vi "MARS_SiPM_Data_Analysis.vi"() -> ()   [LabVIEW 2015]
uses:
  <vilib>/Utility/tdmsutil.llb/fileViewerConfigData.ctl
  Data_Analysis_subvis/ESA_Data_Analysis_Global_VIs.vi
  <vilib>/Analysis/NI_AALPro.lvlib
panel:
  in  "Add Chs":bool
  in  "Offset":dbl=-7.5e-05 step=1e-05 format="%#.3p"
  in  "Discr. Slope":dbl=3.07 min=0.0 step=0.1 format="%#.3p"
  out "Indicator":bool
  in  "Listbox":i32[](listbox) caption="File Name"
  in  "Contents sel":bool
  in  "Sim. Analysis":bool
  in  "Tab Sel 2":enum32{"Radio Selection 1", "Radio Selection 2"}(radio)
  in  "Analysis tab":enum32{"Analysis", "Spectrum"}(tab)
  out "Intensity Graph":u32[][](graph)
  out "Histogram":u32[](graph)
  in  "Graph sel":bool=TRUE
  out "Scatter Plot":cluster{"Array":dbl[], "Array":dbl[]}[](graph)
  in  "File Vs Discr":bool
  in  "PeakVs Integral":bool
  out "Spectrum":T1(graph)
  in  "# bins":i32=256
  in  "Max":dbl=0.2 format="%#.3p"
  in  "Min":dbl format="%#.3p"
  out "Nb of Neutron Counts":i32
  out "Nb of Gamma Counts":i32
  out "Total Counts":i32
  in  "Tab Sel":T2(radio)
  in  "Data tab":enum32{"Raw", "Filtered", "Properties"}(tab)
  out "Boolean 2":bool
  out "Boolean":bool
  in  "Nb of Samples as Offset":i32=50
  in  "Display sel":bool
  out "SiPM Waveform":waveform(dbl)[](graph)
  out "Total Int.":dbl caption="Total Integration Duration (s)" format="%#.3p"
  out "Tail Int.":dbl caption="Tail Integration Duration (s)" format="%#.3p"
  in  "Nb of Samples to Display":i32=50
  out "T3b (s)":dbl format="%#.3p"
  out "T2b (s)":dbl format="%#.3p"
  out "T1b (s)":dbl format="%#.3p"
  out "T3a (s)":dbl format="%#.3p"
  out "T2a (s)":dbl format="%#.3p"
  out "T1a (s)":dbl format="%#.3p"
  out "Table":string[][](table)
  in  "Std Dev 3":dbl=0.005 format="%0.2f"
  in  "Std Dev 2":dbl=0.04 format="%0.2f"
  in  "Graph resolution":dbl=5.0
  in  "Com. std dev":dbl=0.4 format="%0.2f"
  in  "Create Graph":bool
  in  "Nb of smpls":i32=10 min=0 max=50000
  in  "Stop Button":bool
  in  "Open Button":bool
  out "Spectrum Data":T3
  out "Integral Spectrum":dbl[][](array[numeric])
  out "Bins cluster":cluster{"Max":dbl, "Min":dbl, "# bins":i32}
  out "Discr. Slope":cluster{"Array":dbl[], "Array":dbl[]}
  out "Scatter Data":cluster{"Array":dbl[], "Array":dbl[]}
  out "Nb of Channels in Group":i32
  out "Array 2":dbl[](array[numeric])
  out "Array 1":dbl[](array[numeric])
  out "dt":dbl
  out "Total Integral":dbl[](array[numeric])
  out "Tail Integral":dbl[](array[numeric])
  out "group names":string[](array[string])
  out "tdms file out":refnum<k34>
  in  "File contents":string[](tree)
  # "MARS  SiPM Characterization"
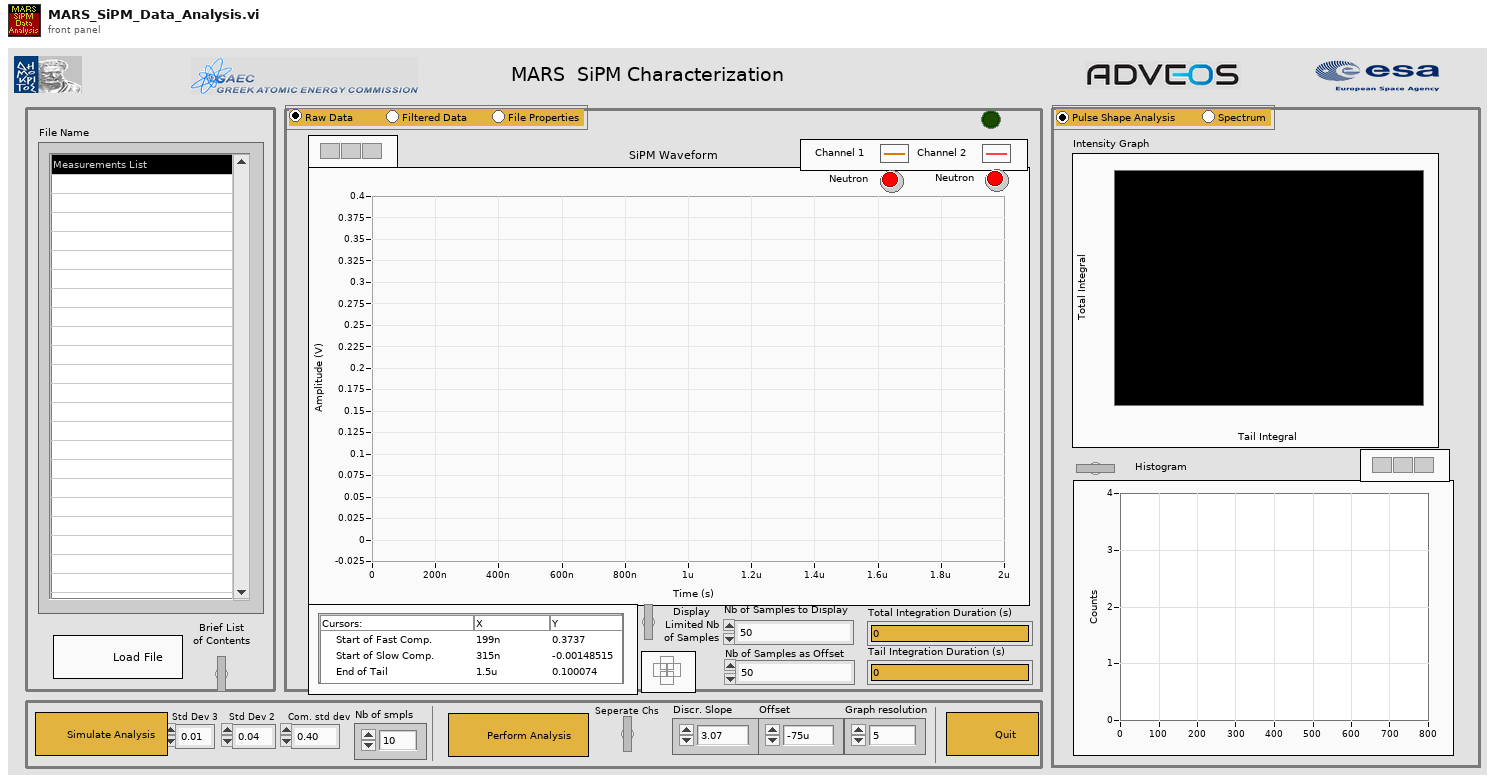
[diagram p1: front panel]
types:
  T1 = cluster{"X Values":dbl[], "Histogram: h(x)":i32[]}[]
  T2 = enum32{"Radio Selection 1", "Radio Selection 2", "Radio Selection 3"}
  T3 = cluster{"Gamma Spectrum":dbl[], "Gamma Integral":dbl[], "Neutron Spectrum":dbl[], "Neutron Integral":dbl[]}
  T4 = typedef "fileViewerConfigData.ctl" = cluster{"Show all (table)":bool, "Show all (graph)":bool, "limit (table)":u64, "limit (graph)":u64, "no show":bool, "start (table)":u64, "start (graph)":u64}
  T5 = enum16{"open", "open or create", "create or replace", "create", "open (read-only)"}
  T6 = cluster{"Cursor.Cursor X":dbl, "Cursor.Cursor Y":dbl, "Cursor.Cursor X":dbl, "Cursor.Cursor Y":dbl}
  T7 = cluster{"X Values":dbl[], "Histogram: h(x)":i32[]}
  T8 = cluster{"Numeric Control":i32, "Numeric Control":i32, "Numeric Control":i32}
  T9 = cluster{"Scatter Plot":cluster{"Array":dbl[], "Array":dbl[]}, "Intensity graph":u32[][], "Histogram":u32[]}
  T10 = cluster{"Tail Integral":dbl[], "Total Integral":dbl[]}
  T11 = cluster{"Tail Integral":dbl[], "Total Integral":dbl[]}[]
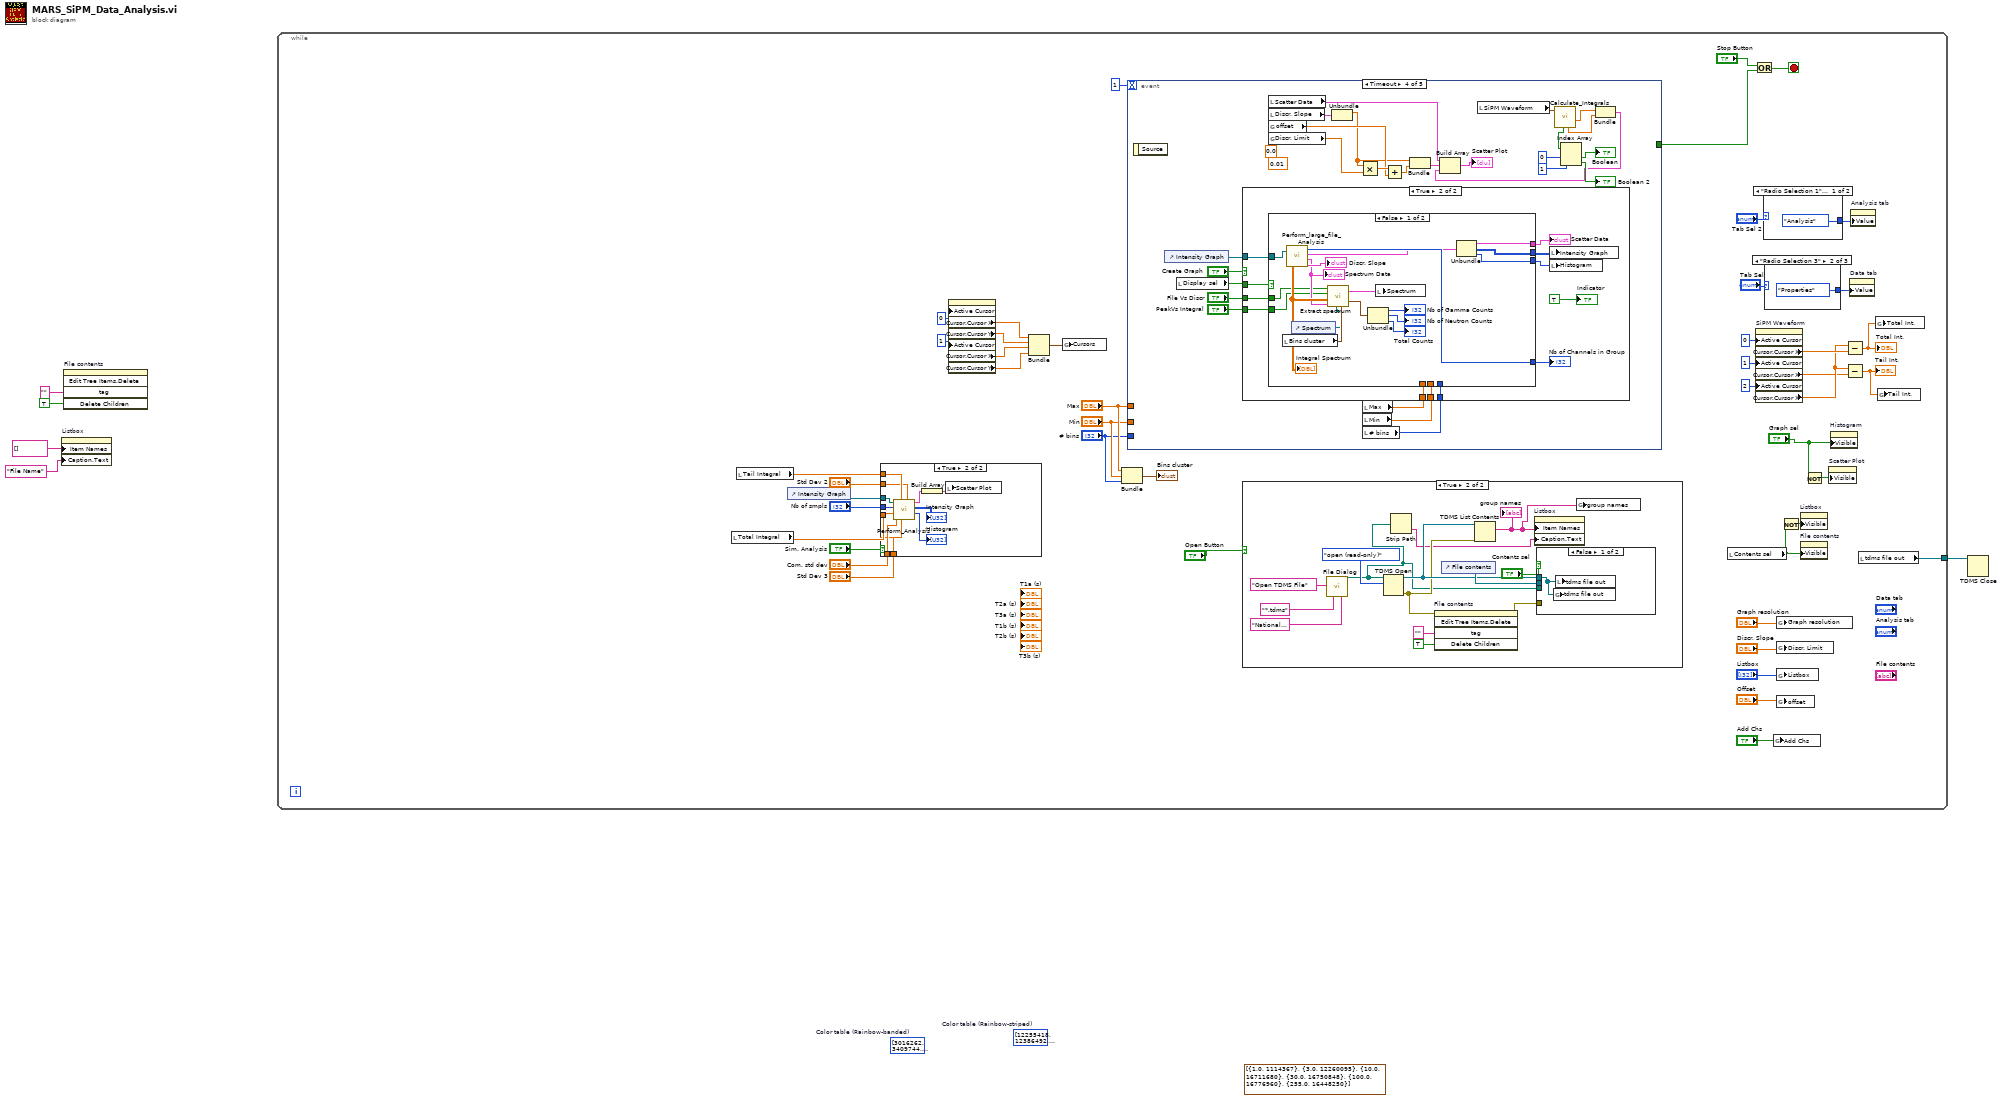
[diagram p0: block diagram]
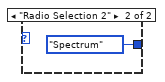
[diagram p2: hidden frame]
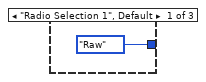
[diagram p3: hidden frame]
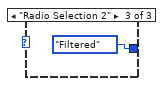
[diagram p4: hidden frame]
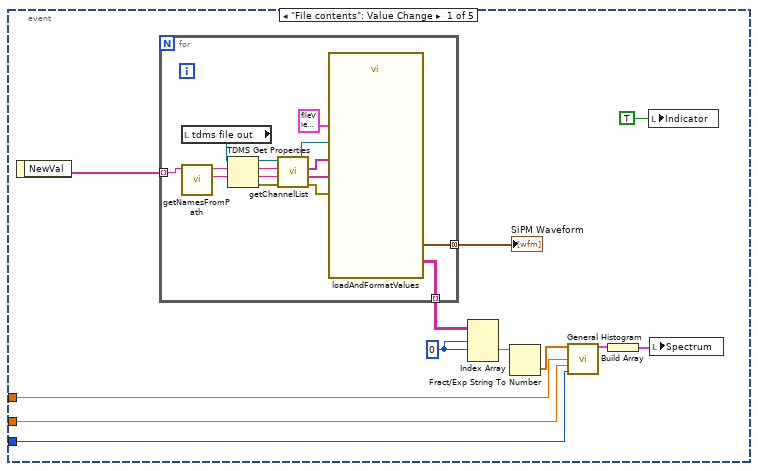
[diagram p6: hidden frame]
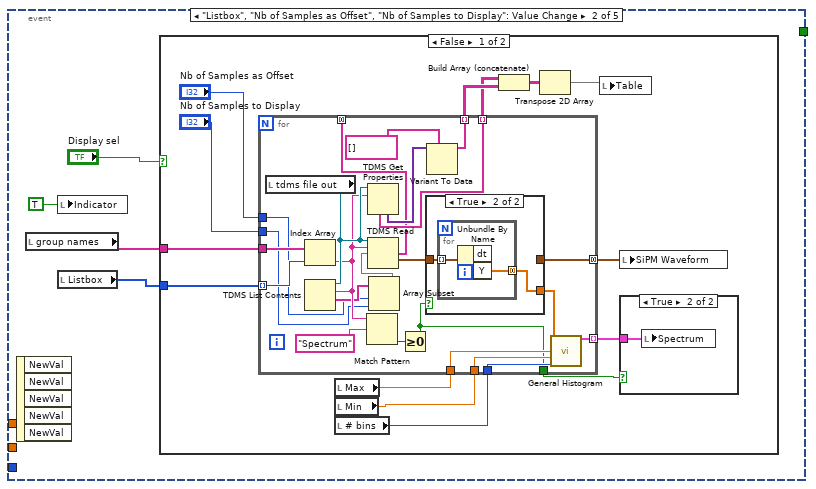
[diagram p7: hidden frame]
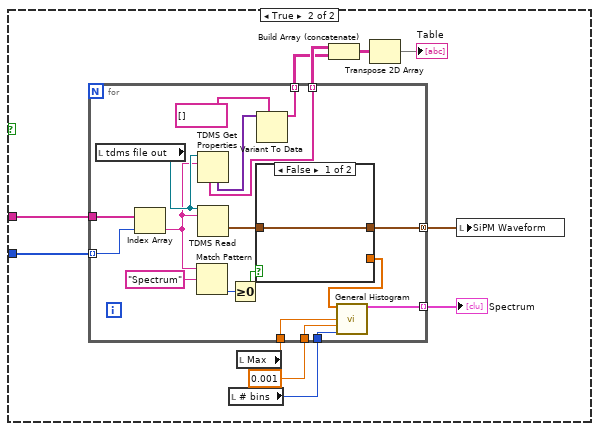
[diagram p10: hidden frame]
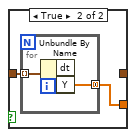
[diagram p11: hidden frame]
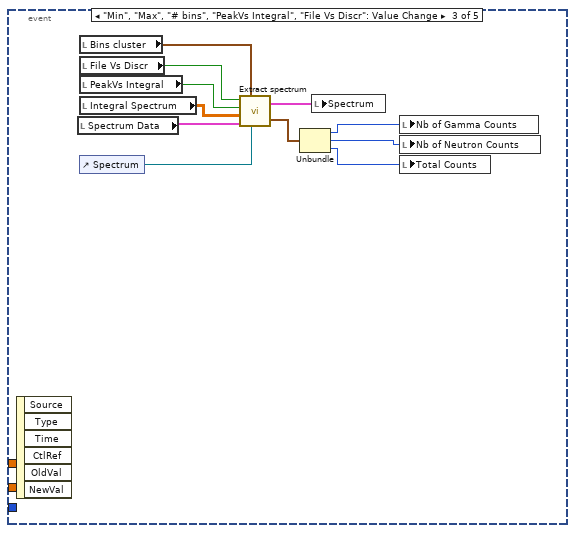
[diagram p12: hidden frame]
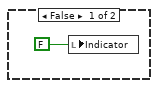
[diagram p13: hidden frame]
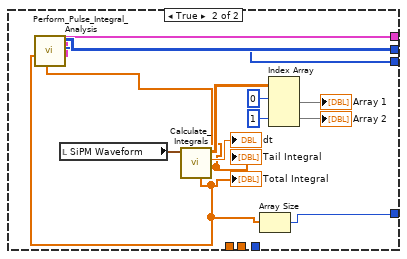
[diagram p14: hidden frame]
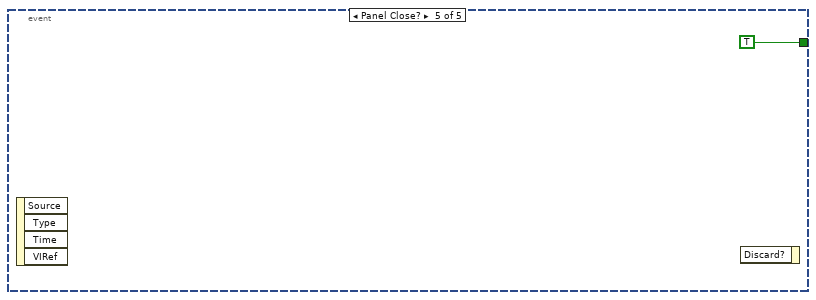
[diagram p15: hidden frame]
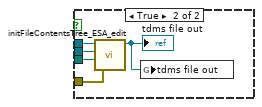
[diagram p17: hidden frame]
diagram:
  (unwired) cluster{dbl, u32}[] [{1.0, 1114367}, {3.0, 12260095}, {10.0, 16711680}, {30.0, 16750848}, {100.0, 16776960}, {255.0, 16448250}] ("Z Scale.Marker Values[]")
  (unwired) u32[] [12255418, 12386492, 12517567, 12320960, 12189888, 12058817, 11927746, 11731139, 11600067, 9175197, 9044125, 11141318, 11010246, 10813639, 10682568, 10551497, 10354890, 10223818, 10092747, 7930019, 7798948, 9633997, 9502926, 9306319, 9175248, 9044176, 8847569, 8716498, 8585427, 6750377, 6619306, 8126677, 7995606, 7798999, 7667927, 7536856, 7340249, 7209178, 7078106, 5505199, 5374128, 6619357, 6488285, 6291678, 6160607, 6029536, 5832929, 5701857, 5570786, 4325557, 4194486, 5112036, 4980965, 4784358, 4653287, 4522215, 4325608, 4194537, 4063466, 3080380, 3014844, 3604716, 3408109, 3277038, 3277038, 3145966, 3014895, 2818288, 2687217, 2556145, 1900738, 1769666, 2097396, 1900789, 1769717, 1638646, 1507575, 1310968, 1179896, 1048825, 721096, 590024, 590075, 393468, 262397, 131326, 255, 1791, 3327, 4863, 5068, 6348, 9471, 11007, 12543, 14079, 15615, 17151, 18687, 20223, 17612, 18636, 25087, 26623, 28159, 29695, 31231, 32767, 34303, 35839, 29900, 31180, 40447, 41983, 43775, 45311, 46847, 48383, 49919, 51455, 42444, 43724, 56063, 57599, 59135, 60671, 62207, 63743, 65535, 65528, 52418, 52413, 65510, 65504, 65498, 65492, 65486, 65480, 65474, 65468, 52369, 52364, 65449, 65443, 65437, 65431, 65425, 65419, 65413, 65407, 52321, 52316, 65389, 65383, 65377, 65371, 65364, 65358, 65352, 65346, 52272, 52267, 65328, 65322, 65316, 65310, 65304, 65298, 65292, 65286, 52224, 314368, 851712, 1244928, 1638144, 2031360, 2424576, 2817792, 3211008, 3604224, 3197952, 3525632, 4783872, 5177088, 5635840, 6029056, 6422272, 6815488, 7208704, 7601920, 6409216, 6736896, 6736896, 8781568, 9174784, 9568000, 9961216, 10354432, 10747648, 11206400, 11599616, 9554944, 9882624, 12779264, 13172480, 13565696, 13958912, 14352128, 14745344, 15138560, 15531776, 12766208, 13093888, 16776960, 16775170, 16773637, 16771847, 16770314, 16768780, 16766991, 16765457, 13411088, 13409810, 16760601, 16758812, 16757278, 16755745, 16753955, 16752422, 16750888, 16749099, 13398052, 13396774, 16744243, 16742704, 16741166, 16739884, 16738345, 16736807, 16735269, 16733730, 13385753, 13384728, 16729371, 16727833, 16726295, 16725012, 16723474, 16721936, 16720397, 16718859, 13373959, 13372677, 16714500, 16712962, 16711680]  # Color table (Rainbow-striped)
  (unwired) u32[] [3016262, 3409744, 4000097, 4721526, 5508493, 6229924, 6820281, 7214025, 7345364, 7279831, 6886611, 6362057, 5640632, 4788132, 4001165, 3214197, 2492769, 2033488, 1640006, 1508930, 1508934, 1640272, 1902945, 2165622, 2428301, 2690980, 2822585, 2888649, 2757844, 2626775, 2299091, 1971145, 1642936, 1249188, 920973, 724086, 592737, 461392, 395846, 396098, 396358, 462928, 595297, 727925, 861069, 994212, 1127608, 1260745, 1328083, 1329111, 1329876, 1264073, 1132217, 999844, 866957, 734070, 600929, 468304, 401734, 401730, 402502, 469584, 603489, 737909, 737909, 872845, 1008036, 1143224, 1277641, 1345747, 1347287, 1347796, 1281225, 1147833, 1013668, 878989, 743798, 609121, 475216, 407878, 407362, 408390, 476496, 611681, 747893, 884877, 1022116, 1158840, 1294793, 1363667, 1365719, 1365202, 1296836, 1161649, 1025178, 888194, 751211, 614742, 479302, 411196, 410168, 411193, 479297, 614732, 750939, 888171, 1025145, 1161350, 1296782, 1364883, 1365906, 1365132, 1296769, 1161588, 1025124, 888147, 751172, 614710, 479276, 411173, 410146, 411170, 479270, 614700, 750900, 888124, 1025091, 1161289, 1296716, 1364813, 1365834, 1365062, 1296703, 1161527, 1025070, 888101, 751133, 614678, 479249, 411149, 410124, 411147, 479244, 614668, 750861, 888078, 1156111, 1488913, 1820947, 2151188, 2414356, 2610196, 2738451, 2668817, 2597903, 2329869, 2061835, 1794313, 1593351, 1459718, 1458694, 1590790, 1921031, 2449673, 3110155, 3902733, 4695055, 5486609, 6211859, 6738708, 7132948, 7197716, 7063827, 6666513, 6136847, 5410061, 4617739, 3957001, 3362823, 2967046, 2900486, 3098118, 3690503, 4546825, 5666059, 6917389, 8233999, 9484305, 10537235, 11326228, 11786004, 11785236, 11785236, 11454739, 10729745, 9675791, 8424717, 7173643, 6054153, 5066759, 4474374, 4342278, 4605190, 5262855, 6380553, 7695883, 9273613, 10785807, 12100625, 13217555, 13874452, 14136340, 13938196, 13214227, 12161553, 10780431, 9267725, 7755531, 6374921, 5257479, 4599814, 4336646, 4599302, 5255943, 6372361, 7685899, 9261837, 10771983, 12085009, 13200659, 13856532, 14118164, 13920276, 13197075, 12145937, 10766351, 9255949, 7745547, 6366729, 5250567, 4593926, 4331014, 4593158, 5249287, 6364169, 7675915, 9249805, 10758159, 12069393, 13183507, 13838612, 14099988, 13902356, 13180179, 12130065, 10752527]  # Color table (Rainbow-banded)
  n1 = property on="Listbox" class="LstBox (strict)"("Item Names"=string[] [], "Caption.Text"="File Name") -> ()  [unwired: 2 in, 2 out]
  n2 = invoke on="File contents" class="Tree (strict)" method="Edit Tree Items.Delete"("tag"="" ("Tag"), "Delete Children"=TRUE ("Delete Children?")) -> ()  [unwired: 3 in, 5 out]
  n3 = while {
    tunnel: [w49] -> w5
    stop <- w26 stop-if-true
    n4 = local read "Total Integral"() -> (w28:dbl[])
    n5 = local read "Tail Integral"() -> (w29:dbl[])
    n6 = control-ref of="Intensity Graph"() -> (w27:refnum<vi>)
    n7 = case shown="True" "Sim. Analysis" {
      tunnel: w29 -> [_ w67]
      tunnel: w28 -> [_ w66]
      tunnel: "Com. std dev" -> [_ w63]
      tunnel: "Std Dev 3" -> [_ w62]
      tunnel: "Std Dev 2" -> [_ w61]
      tunnel: w27 -> [_ w60]
      tunnel: "Nb of smpls" -> [_ w59]
      frame False {
      }
      frame True {
        n8 = call "Perform_Analysis.vi"("Std Dev in"=w61, "Std Dev 3"=w62, "Array 2"=w67, "Common std dev"=w63, "Array"=w66, "Nb of samples"=w59, "IntensityGraph in"=w60) -> ("Histogram"=→"Histogram":u32[], "Intensity Graph"=→"Intensity Graph":u32[][], "Scatter Plot"=w58:cluster{dbl[], dbl[]})  [unwired: 2 in]
        n9 = Build Array(w58) -> (w57:cluster{dbl[], dbl[]}[])
        n10 = local write "Scatter Plot"(w57) -> ()
      }
    }
    n11 = property on="SiPM Waveform" class="WFGraph (strict)"("Active Cursor"=u32 0, "Active Cursor"=u32 1) -> ("Cursor.Cursor X"=w21:dbl, "Cursor.Cursor Y"=w20:dbl, "Cursor.Cursor X"=w19:dbl, "Cursor.Cursor Y"=w18:dbl)  [unwired: 2 in, 2 out]
    n12 = Bundle("Cursor.Cursor X"=w21, "Cursor.Cursor Y"=w20, "Cursor.Cursor X"=w19, "Cursor.Cursor Y"=w18) -> (w13:T6)  [unwired: 1 in]
    n13 = global write "ESA_Data_Analysis_Global_VIs.vi" "Cursors"(w13) -> ()
    n14 = Bundle("Max"="Max", "Min"="Min", "# bins"="# bins") -> (→"Bins cluster":cluster{"Max":dbl, "Min":dbl, "# bins":i32})  [unwired: 1 in]
    n15 = event shown="[3] Timeout" {
      selector: _ -> [_ _ _ _ _]
      dyn-events: _ -> [_ _ _ _ _]
      timeout: 1 -> [_ _ _ _ _]
      tunnel: [_ _ _ _ TRUE ("Stop Button")] -> w25
      tunnel: "Max" -> [w70 _ _ _ _]
      tunnel: "Min" -> [w69 _ _ _ _]
      tunnel: "# bins" -> [w68 _ _ _ _]
      event "File contents": Value Change {
        w76 = 0 ("disabled index (col)")
        n16 = event-data() -> ("NewVal"=w79:string[])  [unwired: 1 in]
        n17 = for {
          tunnel: [w81] -> w78 mode=concatenating
          tunnel: w79 -> [w82] mode=indexing
          tunnel: [w80] -> w77 mode=indexing
          n18 = local read "tdms file out"() -> (w88:refnum<k34>)
          n19 = call <vilib>:"getNamesFromPath.vi"("tree path"=w82) -> ("channel"=w89:string, "group"=w90:string)  [unwired: 1 in, 4 out]
          n20 = TDMS Get Properties(9:w89, 10:w90, 11:w88) -> (0:w93:errorcluster, 1:w92:string, 2:w91:string, 3:w94:refnum<k34>)  [unwired: 1 in, 4 out]
          n21 = call <vilib>:"getChannelList.vi"("error in (no error)"=w93, "channel names"=w92, "group name"=w91, "tdms file"=w94) -> ("error out"=w85:errorcluster, "channel names out"=w86:string[], "group names out"=w87:string[], "tdms file out"=w84:refnum<k34>)
          n22 = call <vilib>:"loadAndFormatValues.vi"("error in (no error)"=w85, "configuration"=T4 {"Show all (table)"=TRUE, "Show all (graph)"=TRUE, "limit (table)"=0, "limit (graph)"=0, "no show"=FALSE, "start (table)"=0, "start (graph)"=0}, "channel names"=w86, "group names"=w87, "tdms file"=w84) -> ("waveform values"=w81:waveform(dbl)[], "table values"=w80:string[][])  [unwired: 5 out]
        }
        "SiPM Waveform" <- w78
        n23 = Index Array(array=w77, index (dim 0)=w76, index (dim 1)=w76) -> (element=w75:string[])  [unwired: 1 in]
        n24 = Fract/Exp String To Number(string=w75) -> (number=w74:dbl[])  [unwired: 3 in, 1 out]
        n25 = call <vilib>:"General Histogram.vi"("X"=w74, "max"=w70, "min"=w69, "# bins"=w68) -> ("Histogram Graph"=w73:T7)  [unwired: 7 in, 4 out]
        n26 = Build Array(w73) -> (w72:T1)
        n27 = local write "Indicator"(TRUE ("Indicator")) -> ()
        n28 = local write "Spectrum"(w72) -> ()
      }
      event "Listbox", "Nb of Samples as Offset", "Nb of Samples to Display": Value Change {
        n29 = event-data() -> ()  [unwired: 1 in, 5 out]
        n30 = local read "group names"() -> (w98:string[])
        n31 = local write "Indicator"(TRUE ("Indicator")) -> ()
        n32 = local read "Listbox"() -> (w97:i32[])
        n33 = case shown="False" "Display sel" {
          tunnel: w98 -> [w112 w152]
          tunnel: w97 -> [w111 w147]
          frame False {
            n34 = local read "Max"() -> (w109:dbl)
            n35 = local read "Min"() -> (w101:dbl)
            n36 = local read "# bins"() -> (w110:i32)
            n37 = for {
              tunnel: w112 -> [w136]
              tunnel: w111 -> [w135] mode=indexing
              tunnel: [w131] -> w108 mode=concatenating
              tunnel: w109 -> [w130]
              tunnel: w101 -> [w129]
              tunnel: w110 -> [w128]
              tunnel: [w126] -> w103 mode=indexing
              tunnel: [w125] -> w105 mode=indexing
              tunnel: [w123] -> w106 mode=indexing
              tunnel: "Nb of Samples to Display" -> [w118]
              tunnel: "Nb of Samples as Offset" -> [w116]
              tunnel: [w115] -> _ mode=concatenating
              tunnel: [w114] -> w99
              n38 = local read "tdms file out"() -> (w121:refnum<k34>)
              n39 = Index Array(array=w136, index=w135) -> (element=w120:string)
              n40 = TDMS List Contents(6:w120, 7:w121) -> (1:w119:string[])  [unwired: 1 in, 3 out]
              n41 = Match Pattern(string=w120, regular expression="Spectrum") -> (offset past match=w133:i32)  [unwired: 1 in, 3 out]
              n42 = TDMS Get Properties(10:w120, 11:w121) -> (4:w122:variant[], 6:w125:string[])  [unwired: 4 in, 4 out]
              n43 = Array Subset(array=w119, index=w116, length=w118) -> (w117:string[])
              n44 = TDMS Read(0:w121, 5:w120, 7:w117) -> (8:w115:string[], 10:w132:waveform(dbl)[])  [unwired: 5 in, 4 out]
              n45 = Greater Or Equal To 0?(x=w133) -> (x >= 0?=w114:bool)
              n46 = case shown="True" w114 {
                tunnel: [_ w139] -> w127
                tunnel: w132 -> [w137 w138]
                tunnel: [w137 _] -> w131
                frame False {
                }
                frame True {
                  n47 = for {
                    tunnel: [w141] -> w139 mode=concatenating
                    tunnel: w138 -> [w140] mode=indexing
                    n48 = Unbundle By Name(w140) -> ("Y"=w141:dbl[])  [unwired: 1 out]
                  }
                }
              }
              n49 = Variant To Data(type=string[] [] ("property names"), Variant=w122) -> (data=w123:string[])  [unwired: 1 in, 1 out]
              n50 = call <vilib>:"General Histogram.vi"("X"=w127, "max"=w130, "min"=w129, "# bins"=w128) -> ("Histogram Graph"=w126:T7)  [unwired: 7 in, 4 out]
            }
            n51 = Build Array (concatenate)(w105, w106) -> (w107:string[][])
            n52 = Transpose 2D Array(2D array=w107) -> (transposed array=w104:string[][])
            n53 = local write "Table"(w104) -> ()
            n54 = local write "SiPM Waveform"(w108) -> ()
            n55 = case shown="True" w99 {
              tunnel: w103 -> [_ w113]
              frame False {
              }
              frame True {
                n56 = local write "Spectrum"(w113) -> ()
              }
            }
          }
          frame True {
            n57 = local read "# bins"() -> (w149:i32)
            n58 = local read "Max"() -> (w151:dbl)
            n59 = for {
              tunnel: w152 -> [w170]
              tunnel: w147 -> [w169] mode=indexing
              tunnel: [w165] -> w142 mode=concatenating
              tunnel: w151 -> [w164]
              tunnel: 0.001 ("min") -> [w163]
              tunnel: w149 -> [w162]
              tunnel: [w160] -> w148 mode=indexing
              tunnel: [w156] -> w144 mode=indexing
              tunnel: [w154] -> w143 mode=indexing
              n60 = local read "tdms file out"() -> (w158:refnum<k34>)
              n61 = Index Array(array=w170, index=w169) -> (element=w157:string)
              n62 = Match Pattern(string=w157, regular expression="Spectrum") -> (offset past match=w167:i32)  [unwired: 1 in, 3 out]
              n63 = TDMS Get Properties(10:w157, 11:w158) -> (4:w153:variant[], 6:w156:string[])  [unwired: 4 in, 4 out]
              n64 = TDMS Read(0:w158, 5:w157) -> (10:w166:waveform(dbl)[])  [unwired: 6 in, 5 out]
              n65 = Greater Or Equal To 0?(x=w167) -> (x >= 0?=w159:bool)
              n66 = case shown="False" w159 {
                tunnel: [_ w173] -> w161
                tunnel: w166 -> [w171 w172]
                tunnel: [w171 _] -> w165
                frame False {
                }
                frame True {
                  n67 = for {
                    tunnel: [w175] -> w173 mode=concatenating
                    tunnel: w172 -> [w174] mode=indexing
                    n68 = Unbundle By Name(w174) -> ("Y"=w175:dbl[])  [unwired: 1 out]
                  }
                }
              }
              n69 = Variant To Data(type=string[] [] ("property names"), Variant=w153) -> (data=w154:string[])  [unwired: 1 in, 1 out]
              n70 = call <vilib>:"General Histogram.vi"("X"=w161, "max"=w164, "min"=w163, "# bins"=w162) -> ("Histogram Graph"=w160:T7)  [unwired: 7 in, 4 out]
            }
            "Spectrum" <- w148
            n71 = Build Array (concatenate)(w144, w143) -> (w146:string[][])
            n72 = Transpose 2D Array(2D array=w146) -> (transposed array=→"Table":string[][])
            n73 = local write "SiPM Waveform"(w142) -> ()
          }
        }
      }
      event "Min", "Max", "# bins", "PeakVs Integral", "File Vs Discr": Value Change {
        n74 = event-data() -> ()  [unwired: 1 in, 6 out]
        n75 = local read "Spectrum Data"() -> (w182:T3)
        n76 = local read "Bins cluster"() -> (w186:cluster{"Max":dbl, "Min":dbl, "# bins":i32})
        n77 = local read "File Vs Discr"() -> (w180:bool)
        n78 = local read "PeakVs Integral"() -> (w181:bool)
        n79 = local read "Integral Spectrum"() -> (w183:dbl[][])
        n80 = control-ref of="Spectrum"() -> (w176:refnum<vi>)
        n81 = call "Extract spectrum.vi"("Spectrum ref"=w176, "Bins Cluster"=w186, "Spectrum Data"=w182, "Integral Spectrum"=w183, "Peak Vs Integral"=w181, "File Vs Discr."=w180) -> ("Nb of Counts"=w184:T8, "Spectrum Histogram"=w185:T1)
        n82 = Unbundle(w184) -> ("Numeric Control"=w179:i32, "Numeric Control"=w178:i32, "Numeric Control"=w177:i32)
        n83 = local write "Spectrum"(w185) -> ()
        n84 = local write "Nb of Gamma Counts"(w179) -> ()
        n85 = local write "Nb of Neutron Counts"(w178) -> ()
        n86 = local write "Total Counts"(w177) -> ()
      }
      event Timeout {
        (unwired) 0.0 ("element")
        (unwired) 0.01 ("element")
        n87 = event-data() -> ()  [unwired: 1 in, 1 out]
        n88 = control-ref of="Intensity Graph"() -> (w207:refnum<vi>)
        n89 = local read "Display sel"() -> (w212:bool)
        n90 = local read "Scatter Data"() -> (w194:cluster{"Array":dbl[], "Array":dbl[]})
        n91 = local read "Discr. Slope"() -> (w193:cluster{"Array":dbl[], "Array":dbl[]})
        n92 = global read "ESA_Data_Analysis_Global_VIs.vi" "Discr. Limit"() -> (w205:dbl)
        n93 = global read "ESA_Data_Analysis_Global_VIs.vi" "offset"() -> (w201:dbl)
        n94 = Unbundle(w193) -> ("Array"=w192:dbl[])  [unwired: 1 out]
        n95 = Multiply(x=w192, y=w205) -> (x*y=w206:dbl[])
        n96 = local read "Max"() -> (w210:dbl)
        n97 = local read "Min"() -> (w209:dbl)
        n98 = local read "# bins"() -> (w208:i32)
        n99 = case shown="True" "Create Graph" {
          tunnel: w212 -> [_ w225]
          tunnel: w210 -> [_ w220]
          tunnel: w209 -> [_ w219]
          tunnel: w208 -> [_ w218]
          tunnel: w207 -> [_ w217]
          tunnel: "PeakVs Integral" -> [_ w215]
          tunnel: "File Vs Discr" -> [_ w214]
          frame False {
            n100 = local write "Indicator"(FALSE ("Boolean")) -> ()
          }
          frame True {
            n101 = case shown="False" w225 {
              tunnel: [w240 w249] -> w222
              tunnel: [w239 w248] -> w221
              tunnel: [w241 w247] -> w216
              tunnel: [w243 w244] -> w223
              tunnel: w220 -> [_ _]
              tunnel: w219 -> [_ _]
              tunnel: w218 -> [_ _]
              tunnel: w217 -> [w238 _]
              tunnel: w215 -> [w228 _]
              tunnel: w214 -> [w227 _]
              frame False {
                n102 = local read "Bins cluster"() -> (w235:cluster{"Max":dbl, "Min":dbl, "# bins":i32})
                n103 = call "Perform_large_file_Analysis.vi"("IntensityGraph in"=w238) -> ("Integral Spectrum"=w236:dbl[][], "size(s)"=w243:i32, "Analysis_Data"=w242:T9, "Spectrum Data"=w234:T3, "Discr. Slope"=→"Discr. Slope":cluster{"Array":dbl[], "Array":dbl[]})
                "Integral Spectrum" <- w236
                "Spectrum Data" <- w234
                n104 = control-ref of="Spectrum"() -> (w226:refnum<vi>)
                n105 = call "Extract spectrum.vi"("Spectrum ref"=w226, "Bins Cluster"=w235, "Spectrum Data"=w234, "Integral Spectrum"=w236, "Peak Vs Integral"=w228, "File Vs Discr."=w227) -> ("Nb of Counts"=w232:T8, "Spectrum Histogram"=w233:T1)
                n106 = Unbundle(w232) -> ("Numeric Control"=→"Nb of Gamma Counts":i32, "Numeric Control"=→"Nb of Neutron Counts":i32, "Numeric Control"=→"Total Counts":i32)
                n107 = local write "Spectrum"(w233) -> ()
                n108 = Unbundle(w242) -> ("Scatter Plot"=w241:cluster{"Array":dbl[], "Array":dbl[]}, "Intensity graph"=w240:u32[][], "Histogram"=w239:u32[])
              }
              frame True {
                n109 = local read "SiPM Waveform"() -> (w251:waveform(dbl)[])
                n110 = call "Calculate_Integrals.vi"("SiPM Waveform"=w251) -> ("Tail Integral"=w246:dbl[], "dt"=→"dt":dbl, "Data Points"=w252:dbl[][], "Total Integral"=w245:dbl[])  [unwired: 5 in, 2 out]
                "Tail Integral" <- w246
                "Total Integral" <- w245
                n111 = call "Perform_Pulse_Integral_Analysis.vi"("Tail Integral"=w246, "Total Integral"=w245) -> ("Scatter plot"=w247:cluster{"Array":dbl[], "Array":dbl[]}, "Histogram"=w248:u32[], "Intensity graph"=w249:u32[][])  [unwired: 7 in]
                n112 = Array Size(array=w245) -> (size(s)=w244:i32)
                n113 = Index Array(array=w252, index (row) #1=0 ("index (row)"), index (row) #2=1 ("index (row)")) -> (element #1=→"Array 1":dbl[], element #2=→"Array 2":dbl[])  [unwired: 2 in]
              }
            }
            "Nb of Channels in Group" <- w223
            "Scatter Data" <- w216
            n114 = local write "Intensity Graph"(w222) -> ()
            n115 = local write "Histogram"(w221) -> ()
            "Indicator" <- TRUE ("Boolean")
          }
        }
        n116 = Add(x=w206, y=w201) -> (x+y=w202:dbl[])
        n117 = Bundle("Array"=w192, w202) -> (w204:cluster{"Array":dbl[], dbl[]})  [unwired: 1 in]
        n118 = local read "SiPM Waveform"() -> (w200:waveform(dbl)[])
        n119 = call "Calculate_Integrals.vi"("SiPM Waveform"=w200) -> ("Tail Integral"=w191:dbl[], "Total Integral"=w190:dbl[], "Discrimination boolean"=w199:bool[])  [unwired: 5 in, 3 out]
        n120 = Index Array(array=w199, index #1=0 ("index"), index #2=1 ("index")) -> (element #1=→"Boolean":bool, element #2=→"Boolean 2":bool)
        n121 = Bundle("Tail Integral"=w191, "Total Integral"=w190) -> (w189:T10)  [unwired: 1 in]
        n122 = Build Array(w194, w204, w189) -> (→"Scatter Plot":T11)
      }
      event Panel Close? {
        n123 = event-data() -> ()  [unwired: 1 in, 4 out]
        n124 = event-data() -> ()  [unwired: 2 in, 1 out]
      }
    }
    n125 = case shown="True" "Open Button" {
      frame False {
      }
      frame True {
        n126 = call "File Dialog"("prompt"="Open TDMS File" ("prompt tdms"), "pattern (all files)"="*.tdms", "pattern label"="National Instruments TDM Streaming" ("pattern label tdms")) -> ("selected path"=w260:path)  [unwired: 4 in, 8 out]
        n127 = TDMS Open(10:T5."open (read-only)" ("operation (0:open)"), 11:w260) -> (0:w262:errorcluster, 3:w263:refnum<k34>)  [unwired: 5 in]
        n128 = Strip Path(path=w260) -> (name=w259:string)  [unwired: 1 out]
        n129 = invoke on="File contents" class="Tree (strict)" method="Edit Tree Items.Delete"(error in=w262, "tag"="" ("Tag"), "Delete Children"=TRUE ("Delete Children?")) -> (error out=w270:errorcluster)  [unwired: 2 in, 4 out]
        n130 = control-ref of="File contents"() -> (w271:refnum<vi>)
        n131 = TDMS List Contents(4:w262, 7:w263) -> (2:w258:string[])  [unwired: 1 in, 3 out]
        "group names" <- w258
        n132 = property on="Listbox" class="LstBox (strict)"("Item Names"=w258, "Caption.Text"=w259) -> ()  [unwired: 2 in, 2 out]
        n133 = case shown="False" "Contents sel" {
          tunnel: w271 -> [_ w277]
          tunnel: w270 -> [_ w276]
          tunnel: w260 -> [_ w275]
          tunnel: w263 -> [w272 w274]
          frame False {
            n134 = global write "ESA_Data_Analysis_Global_VIs.vi" "tdms file out"(w272) -> ()
            n135 = local write "tdms file out"(w272) -> ()
          }
          frame True {
            n136 = call "initFileContentsTree_ESA_edit.vi"("error in (no error)"=w276, "file path"=w275, "Tree Refnum"=w277, "tdms file"=w274) -> ("tdms file out"=w273:refnum<k34>)  [unwired: 2 in, 1 out]
            "tdms file out" <- w273
            n137 = global write "ESA_Data_Analysis_Global_VIs.vi" "tdms file out"(w273) -> ()
          }
        }
        n138 = global write "ESA_Data_Analysis_Global_VIs.vi" "group names"(w258) -> ()
      }
    }
    n139 = local read "Contents sel"() -> (w31:bool)
    n140 = Or(x="Stop Button", y=w25) -> (x .or. y?=w26:bool)
    n141 = property on="SiPM Waveform" class="WFGraph (strict)"("Active Cursor"=u32 0, "Active Cursor"=u32 1, "Active Cursor"=u32 2) -> ("Cursor.Cursor X"=w45:dbl, "Cursor.Cursor X"=w43:dbl, "Cursor.Cursor X"=w44:dbl)  [unwired: 2 in, 2 out]
    n142 = case shown="\"Radio Selection 1\", Default" "Tab Sel 2" {
      tunnel: [enum32{"Analysis", "Spectrum"}."Analysis" ("Analysis tab") enum32{"Analysis", "Spectrum"}."Spectrum" ("Analysis tab")] -> w37
      frame "Radio Selection 1", Default {
      }
      frame "Radio Selection 2" {
      }
    }
    n143 = case shown="\"Radio Selection 3\"" "Tab Sel" {
      tunnel: [enum32{"Raw", "Filtered", "Properties"}."Raw" ("Raw data") enum32{"Raw", "Filtered", "Properties"}."Properties" ("Raw data") enum32{"Raw", "Filtered", "Properties"}."Filtered" ("Raw data")] -> w39
      frame "Radio Selection 1", Default {
      }
      frame "Radio Selection 3" {
      }
      frame "Radio Selection 2" {
      }
    }
    n144 = global write "ESA_Data_Analysis_Global_VIs.vi" "Add Chs"("Add Chs") -> ()
    n145 = global write "ESA_Data_Analysis_Global_VIs.vi" "Graph resolution"("Graph resolution") -> ()
    n146 = global write "ESA_Data_Analysis_Global_VIs.vi" "Discr. Limit"("Discr. Slope") -> ()
    n147 = global write "ESA_Data_Analysis_Global_VIs.vi" "Listbox"("Listbox") -> ()
    n148 = global write "ESA_Data_Analysis_Global_VIs.vi" "offset"("Offset") -> ()
    n149 = Not(x=w31) -> (.not. x?=w30:bool)
    n150 = property on="Listbox" class="LstBox (strict)"("Visible"=w30) -> ()  [unwired: 2 in, 2 out]
    n151 = property on="File contents" class="Tree (strict)"("Visible"=w31) -> ()  [unwired: 2 in, 2 out]
    n152 = Not(x="Graph sel") -> (.not. x?=w41:bool)
    n153 = property on="Scatter Plot" class="XYGraph (strict)"("Visible"=w41) -> ()  [unwired: 2 in, 2 out]
    n154 = property on="Histogram" class="WFGraph (strict)"("Visible"="Graph sel") -> ()  [unwired: 2 in, 2 out]
    n155 = Subtract(x=w44, y=w45) -> (x-y=w16:dbl)
    "Total Int." <- w16
    n156 = Subtract(x=w44, y=w43) -> (x-y=w15:dbl)
    "Tail Int." <- w15
    n157 = property on="Data tab" class="TabCtl (strict)"("Value"=w39) -> ()  [unwired: 2 in, 2 out]
    n158 = property on="Analysis tab" class="TabCtl (strict)"("Value"=w37) -> ()  [unwired: 2 in, 2 out]
    n159 = local read "tdms file out"() -> (w49:refnum<k34>)
    n160 = global write "ESA_Data_Analysis_Global_VIs.vi" "Total Int."(w16) -> ()
    n161 = global write "ESA_Data_Analysis_Global_VIs.vi" "Tail Int."(w15) -> ()
  }
  n162 = TDMS Close(11:w5) -> ()  [unwired: 1 in, 2 out]
